vi "execute.vi"(8 "error in (no error)":errorcluster, 11 "command in":refnum<class "command_click.lvclass">) -> (0 "error out":errorcluster, 3 "command out":refnum<class "command_click.lvclass">)   [LabVIEW 2015, in "command_click.lvclass"]
uses:
  canon_m3/command_click.lvclass
  <vilib>/FieldPoint/Polymorphic Write.llb/FP Write (Float Array -IO).vi
  command/command_generic.lvclass
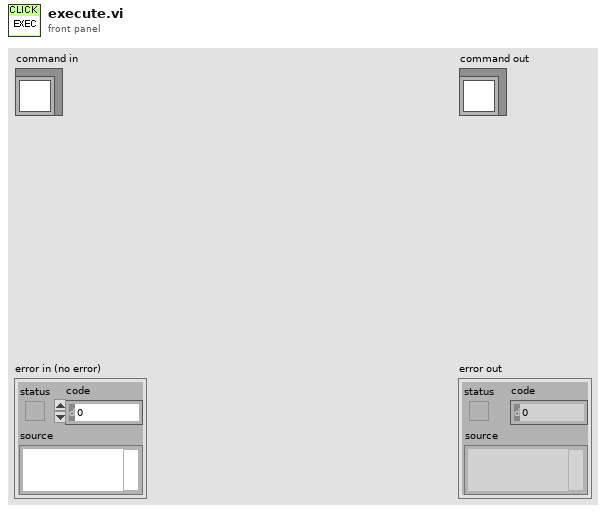
[diagram p1: front panel]
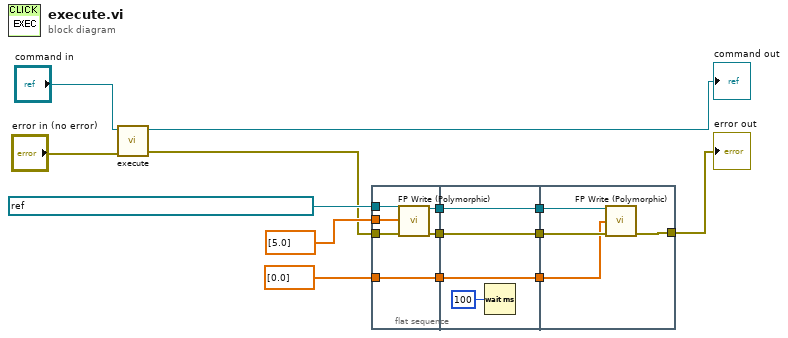
[diagram p0: block diagram]
diagram:
  n1 = call-parent "execute.vi"("error in (no error)"="error in (no error)", "command in"="command in") -> ("error out"=w2:errorcluster, "command out"=→"command out":refnum<class "command_click.lvclass">)  [unwired: 8 in]
  n2 = flat-sequence {
    tunnel: refnum<k21> "sauna_fp\\FP @ 10_0_0_50\\cFP-AIO-610 @1\\Output 0" ("FieldPoint IO Point") -> [w18]
    tunnel: dbl[] [5.0] ("values") -> [w20]
    tunnel: [w19] -> w11
    tunnel: w2 -> [w17]
    tunnel: [w16] -> w10
    tunnel: dbl[] [0.0] ("values") -> [w15]
    tunnel: [w15] -> w9
    tunnel: w11 -> [w23]
    tunnel: [w23] -> w8
    tunnel: [w22] -> w7
    tunnel: w10 -> [w22]
    tunnel: [w21] -> w6
    tunnel: w9 -> [w21]
    tunnel: w8 -> [w28]
    tunnel: w7 -> [w27]
    tunnel: w6 -> [w26]
    tunnel: [w25] -> _
    tunnel: [w25] -> w1
    frame #0 {
      n3 = call-poly <vilib>:"FP Write (Polymorphic).vi"("FieldPoint IO Point In"=w18, "values"=w20, "error in (no error)"=w17) -> ("FieldPoint IO Point Out"=w19:refnum<k21>, "error out"=w16:errorcluster)  [unwired: 10 in, 1 out]
    }
    frame #1 {
      n4 = Wait (ms)(milliseconds to wait=u32 100) -> ()  [unwired: 1 out]
    }
    frame #2 {
      n5 = call-poly <vilib>:"FP Write (Polymorphic).vi"("FieldPoint IO Point In"=w28, "values"=w26, "error in (no error)"=w27) -> ("error out"=w25:errorcluster)  [unwired: 10 in, 2 out]
    }
  }
  "error out" <- w1
